vi "NML SCMPS unpersistence.vi"(5 "VISA session":refnum<visa-resource-name>="GPIB0::22::INSTR") -> (0 "Persistence Out":bool, 1 "String":string, 2 "dup VISA session":refnum<visa-resource-name>)   [LabVIEW 2019]
panel:
  out "Persistence In":bool
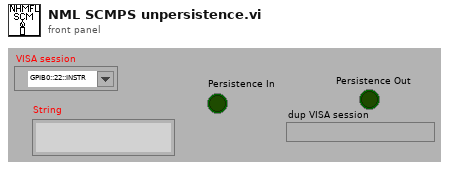
[diagram p1: front panel]
types:
  T1 = enum16{"No Response", "Ramping to programmed field ", "Holding at programmed field", "Paused", "Ramp Manual Up", "Ramp Manual Down", "Ramping to Zero", "QUENCH", "Heating Persistance Switch", "At Zero Current"}
  T2 = enum16{"No Response", "Ramping to programmed field ", "Holding at programmed field", "Paused", "Ramp Manual Up", "Ramp Manual Down", "Ramping to Zero", "QUENCH", "Heating Persistence Switch", "At Zero Current"}
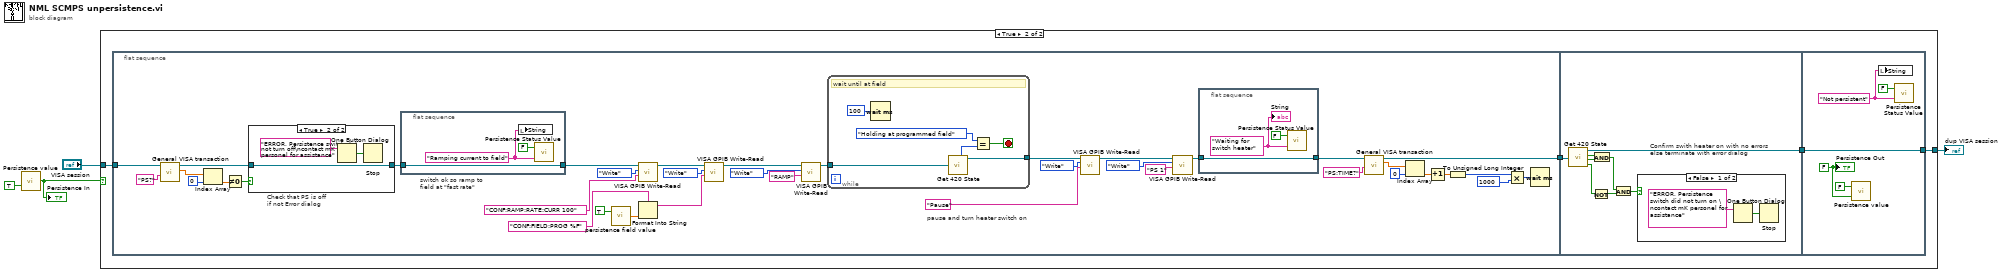
[diagram p0: block diagram]
diagram:
  n1 = call "Persistence value.vi"("Persistence In"=TRUE ("Read/Write")) -> ("Persistence Out"=w2:bool)  [unwired: 1 in]
  "Persistence In" <- w2
  n2 = case shown="True" w2 {
    tunnel: "VISA session" -> [w5 w9]
    tunnel: [w5 w7] -> w1
    frame False {
      # "Not persistent so ignore"
    }
    frame True {
      n3 = flat-sequence {
        tunnel: [w40] -> w8
        tunnel: w9 -> [w16]
        tunnel: w8 -> [w71]
        tunnel: [w64] -> w6
        tunnel: [w74] -> w7
        tunnel: w6 -> [w74]
        frame #0 {
          # "Check that PS is off \nif not Error dialog"
          # "switch ok so ramp to field at \"fast rate\""
          # "pause and turn heater switch on"
          n4 = call "General VISA transaction.vi"("Command String"="PS?", "VISA Session"=w16) -> ("Measurement"=w20:dbl[], "dup VISA Session"=w15:refnum<visa-resource-name>)  [unwired: 4 in, 4 out]
          n5 = Index Array(array=w20, index=0) -> (element=w18:dbl)
          n6 = Not Equal To 0?(x=w18) -> (x != 0?=w17:bool)
          n7 = case shown="True" w17 {
            tunnel: [w48 w49] -> w11
            tunnel: w15 -> [w48 w49]
            frame False {
            }
            frame True {
              n8 = One Button Dialog(message="ERROR, Persistence switch did not turn off\ncontact mK personel for assistance") -> (true=w50:bool)  [unwired: 1 in]
              n9 = Stop(stop? (T)=w50) -> ()
            }
          }
          n10 = flat-sequence {
            tunnel: w11 -> [w52]
            tunnel: [w52] -> w10
            frame #0 {
              w54 = "Ramping current to field" ("String")
              n11 = local write "String"(w54) -> ()
              n12 = call "Persistence Status Value.vi"("Persistence Status In"=w54, "Read/Write this vi"=FALSE) -> ()  [unwired: 1 out]
            }
          }
          n13 = call "persistence field value.vi"("Read/Write this vi"=TRUE) -> ("Persistent Field Out"=w22:dbl)  [unwired: 1 in]
          n14 = call "VISA GPIB Write-Read.vi"("Command"="CONF:RAMP:RATE:CURR 100" ("String to Write"), "Action"=enum16{"Write", "Read", "Write & Read"}."Write", "VISA resource name"=w10) -> ("dup VISA Session"=w30:refnum<visa-resource-name>)  [unwired: 5 in, 3 out]
          n15 = Format Into String(format string="CONF:FIELD:PROG %F" ("Command String"), w22) -> (resulting string=w28:string)  [unwired: 2 in, 1 out]
          n16 = call "VISA GPIB Write-Read.vi"("Command"=w28, "Action"=enum16{"Write", "Read", "Write & Read"}."Write", "VISA resource name"=w30) -> ("dup VISA Session"=w26:refnum<visa-resource-name>)  [unwired: 5 in, 3 out]
          n17 = call "VISA GPIB Write-Read.vi"("Command"="RAMP" ("String to Write"), "Action"=enum16{"Write", "Read", "Write & Read"}."Write", "VISA resource name"=w26) -> ("dup VISA Session"=w33:refnum<visa-resource-name>)  [unwired: 5 in, 3 out]
          n18 = while {
            tunnel: w33 -> [w63]
            tunnel: [w58] -> w34
            stop <- w60 stop-if-true
            # "wait until at field"
            n19 = Wait (ms)(milliseconds to wait=u32 100) -> ()  [unwired: 1 out]
            n20 = call "Get 420 State.vi"("VISA session"=w63) -> ("State"=w62:T2, "dup VISA session"=w58:refnum<visa-resource-name>)  [unwired: 4 out]
            n21 = Equal?(x=T1."Holding at programmed field" ("y"), y=w62) -> (x = y?=w60:bool)
          }
          n22 = call "VISA GPIB Write-Read.vi"("Command"="Pause" ("String to Write"), "Action"=enum16{"Write", "Read", "Write & Read"}."Write", "VISA resource name"=w34) -> ("dup VISA Session"=w37:refnum<visa-resource-name>)  [unwired: 5 in, 3 out]
          n23 = call "VISA GPIB Write-Read.vi"("Command"="PS 1" ("String to Write"), "Action"=enum16{"Write", "Read", "Write & Read"}."Write", "VISA resource name"=w37) -> ("dup VISA Session"=w13:refnum<visa-resource-name>)  [unwired: 5 in, 3 out]
          n24 = flat-sequence {
            tunnel: w13 -> [w55]
            tunnel: [w55] -> w12
            frame #0 {
              w57 = "Waiting for switch heater"
              n25 = call "Persistence Status Value.vi"("Persistence Status In"=w57, "Read/Write this vi"=FALSE) -> ()  [unwired: 1 out]
              "String" <- w57
            }
          }
          n26 = call "General VISA transaction.vi"("Command String"="PS:TIME?", "VISA Session"=w12) -> ("Measurement"=w46:dbl[], "dup VISA Session"=w40:refnum<visa-resource-name>)  [unwired: 4 in, 4 out]
          n27 = Index Array(array=w46, index=0) -> (element=w43:dbl)
          n28 = Increment(x=w43) -> (x+1=w41:dbl)
          n29 = To Unsigned Long Integer(number=w41) -> (unsigned 32bit integer=w14:u32)
          n30 = Multiply(x=w14, y=u32 1000) -> (x*y=w42:u32)
          n31 = Wait (ms)(milliseconds to wait=w42) -> ()  [unwired: 1 out]
        }
        frame #1 {
          # "Confirm swith heater on with no errors\nelse terminate with error dialog"
          n32 = call "Get 420 State.vi"("VISA session"=w71) -> ("dup VISA session"=w64:refnum<visa-resource-name>, "Switch Heater"=w70:bool, "Switch heater \nconfirmed"=w69:bool, "Switch Heater Error"=w68:bool)  [unwired: 2 out]
          n33 = Not(x=w68) -> (.not. x?=w66:bool)
          n34 = And(x=w70, y=w69) -> (x .and. y?=w67:bool)
          n35 = And(x=w67, y=w66) -> (x .and. y?=w65:bool)
          n36 = case shown="False" w65 {
            frame False {
              n37 = One Button Dialog(message="ERROR, Persistence switch did not turn on \ncontact mK personel for assistance") -> (true=w72:bool)  [unwired: 1 in]
              n38 = Stop(stop? (T)=w72) -> ()
            }
            frame True {
            }
          }
        }
        frame #2 {
          w78 = "Not persistent" ("String")
          w77 = FALSE
          n39 = call "Persistence value.vi"("Persistence In"=w77, "Read/Write this vi"=FALSE) -> ()  [unwired: 1 out]
          n40 = local write "String"(w78) -> ()
          n41 = call "Persistence Status Value.vi"("Persistence Status In"=w78, "Read/Write this vi"=FALSE) -> ()  [unwired: 1 out]
          "Persistence Out" <- w77
        }
      }
    }
  }
  "dup VISA session" <- w1
